vi "FPGA_Main.vi"() -> ()   [LabVIEW 2018]
uses:
  Data Def/FPGA_AI ADC IO.ctl
  Data Def/FPGA_AI ADC Loop Data.ctl
  Data Def/FPGA_AI ADC Loop State.ctl
  <vilib>/rvi/Emulation/niFpgaGetClockAttributes.vi
  <vilib>/rvi/Emulation/niFpgaSctlEmulationGetInTimedLoop.vi
  <vilib>/rvi/Emulation/niFpgaEmulationReportErrorSimple.vi
  <vilib>/rvi/Emulation/niFpgaCriticalErrorInLSC.vi
  SubVI/24AIO/AO/AO_FPGA.lvlib
panel:
  in  "AO_Data(U32)":u32
  out "C3 AI Data":i16[](array[numeric])
  out "C2 AI Data":i16[](array[numeric])
  out "C1 AI Data":i16[](array[numeric])
  out "C4 AI Data":i16[](array[numeric])
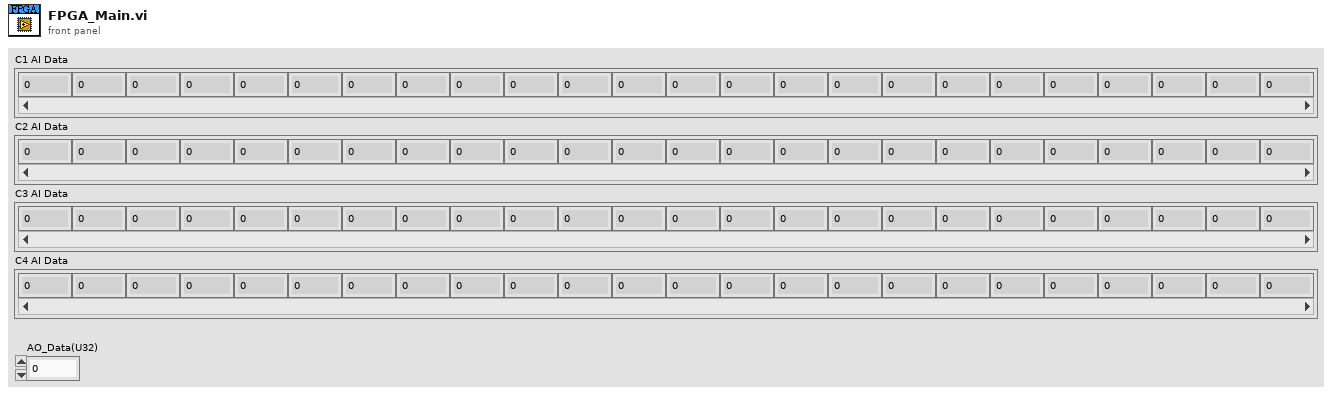
[diagram p1: front panel]
types:
  T1 = cluster{"CS":refnum<k21>, "CLK":refnum<k21>, "MOSI":refnum<k21>}
  T2 = typedef "FPGA_AI ADC IO.ctl" = cluster{"AI_A":cluster{"CONV":refnum<k21>, "RST":refnum<k21>, "SCK":refnum<k21>, "CS":refnum<k21>, "BUSY":refnum<k21>, "DOUT_A":refnum<k21>, "DOUT_B":refnum<k21>, "t_RST (ticks)":u32, "t_CONV (ticks)":u32, "t_BUSYMAX (ticks)":u32}, "AI_B":cluster{"CONV":refnum<k21>, "RST":refnum<k21>, "SCK":refnum<k21>, "CS":refnum<k21>, "BUSY":refnum<k21>, "DOUT_A":refnum<k21>, "DOUT_B":refnum<k21>, "t_RST (ticks)":u32, "t_CONV (ticks)":u32, "t_BUSYMAX (ticks)":u32}, "AI_C":cluster{"CONV":refnum<k21>, "RST":refnum<k21>, "SCK":refnum<k21>, "CS":refnum<k21>, "BUSY":refnum<k21>, "DOUT_A":refnum<k21>, "DOUT_B":refnum<k21>, "t_RST (ticks)":u32, "t_CONV (ticks)":u32, "t_BUSYMAX (ticks)":u32}}
  T3 = typedef "FPGA_AI ADC Loop Data.ctl" = cluster{"AI ADC Loop State":T4, "AI Data":i16[]}
  T4 = typedef "FPGA_AI ADC Loop State.ctl" = enum16{"Initialize", "Get Data"}
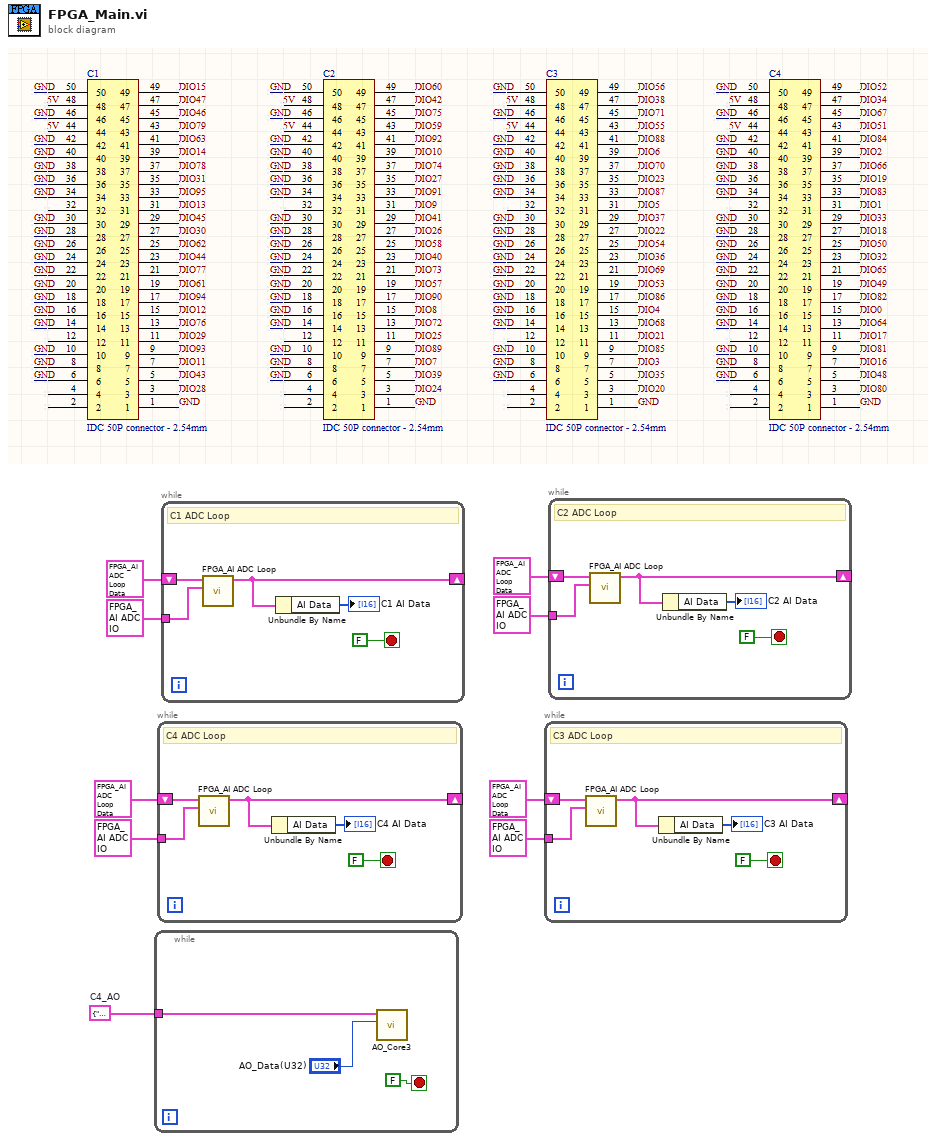
[diagram p0: block diagram]
diagram:
  w1 = T1 {"CS"="RMC/DIO67", "CLK"="RMC/DIO52", "MOSI"="RMC/DIO34"}  # C4_AO
  n1 = while {
    tunnel: w1 -> [w11]
    stop <- FALSE stop-if-true
    n2 = call "AO_Core3.vi"("data"="AO_Data(U32)", "Spi_A"=w11) -> ()  [unwired: 9 in, 1 out]
  }
  n3 = while {
    shift-right: [w17] -> _
    shift-left: T3 {"AI ADC Loop State"=enum."Initialize", "AI Data"=[0, 0, 0, 0, 0, 0, 0, 0, 0, 0, 0, 0, 0, 0, 0, 0, 0, 0, 0, 0, 0, 0, 0, 0]} ("AI ADC Loop Data") -> [w13]
    tunnel: T2 {"AI_A"={"CONV"="RMC/DIO0", "RST"="RMC/DIO64", "SCK"="RMC/DIO17", "CS"="RMC/DIO81", "BUSY"="RMC/DIO16", "DOUT_A"="RMC/DIO48", "DOUT_B"="RMC/DIO80", "t_RST (ticks)"=0, "t_CONV (ticks)"=0, "t_BUSYMAX (ticks)"=0}, "AI_B"={"CONV"="RMC/DIO33", "RST"="RMC/DIO18", "SCK"="RMC/DIO50", "CS"="RMC/DIO32", "BUSY"="RMC/DIO65", "DOUT_A"="RMC/DIO49", "DOUT_B"="RMC/DIO82", "t_RST (ticks)"=0, "t_CONV (ticks)"=0, "t_BUSYMAX (ticks)"=0}, "AI_C"={"CONV"="RMC/DIO51", "RST"="RMC/DIO84", "SCK"="RMC/DIO2", "CS"="RMC/DIO66", "BUSY"="RMC/DIO19", "DOUT_A"="RMC/DIO83", "DOUT_B"="RMC/DIO1", "t_RST (ticks)"=0, "t_CONV (ticks)"=0, "t_BUSYMAX (ticks)"=0}} ("AI ADC IO") -> [w14]
    stop <- FALSE stop-if-true
    # "C4 ADC Loop"
    n4 = call "FPGA_AI ADC Loop.vi"("AI ADC IO"=w14, "AI ADC Loop Data In"=w13) -> ("AI ADC Loop Data Out"=w17:T3)  [unwired: 9 in]
    n5 = Unbundle By Name(w17) -> ("AI Data"=→"C4 AI Data":i16[])
  }
  n6 = while {
    shift-right: [w22] -> _
    shift-left: T3 {"AI ADC Loop State"=enum."Initialize", "AI Data"=[0, 0, 0, 0, 0, 0, 0, 0, 0, 0, 0, 0, 0, 0, 0, 0, 0, 0, 0, 0, 0, 0, 0, 0]} ("AI ADC Loop Data") -> [w18]
    tunnel: T2 {"AI_A"={"CONV"="RMC/DIO12", "RST"="RMC/DIO76", "SCK"="RMC/DIO29", "CS"="RMC/DIO93", "BUSY"="RMC/DIO11", "DOUT_A"="RMC/DIO43", "DOUT_B"="RMC/DIO28", "t_RST (ticks)"=0, "t_CONV (ticks)"=0, "t_BUSYMAX (ticks)"=0}, "AI_B"={"CONV"="RMC/DIO45", "RST"="RMC/DIO30", "SCK"="RMC/DIO62", "CS"="RMC/DIO44", "BUSY"="RMC/DIO77", "DOUT_A"="RMC/DIO61", "DOUT_B"="RMC/DIO94", "t_RST (ticks)"=0, "t_CONV (ticks)"=0, "t_BUSYMAX (ticks)"=0}, "AI_C"={"CONV"="RMC/DIO79", "RST"="RMC/DIO63", "SCK"="RMC/DIO14", "CS"="RMC/DIO78", "BUSY"="RMC/DIO31", "DOUT_A"="RMC/DIO95", "DOUT_B"="RMC/DIO13", "t_RST (ticks)"=0, "t_CONV (ticks)"=0, "t_BUSYMAX (ticks)"=0}} ("AI ADC IO") -> [w19]
    stop <- FALSE stop-if-true
    # "C1 ADC Loop"
    n7 = call "FPGA_AI ADC Loop.vi"("AI ADC IO"=w19, "AI ADC Loop Data In"=w18) -> ("AI ADC Loop Data Out"=w22:T3)  [unwired: 9 in]
    n8 = Unbundle By Name(w22) -> ("AI Data"=→"C1 AI Data":i16[])
  }
  n9 = while {
    shift-right: [w27] -> _
    shift-left: T3 {"AI ADC Loop State"=enum."Initialize", "AI Data"=[0, 0, 0, 0, 0, 0, 0, 0, 0, 0, 0, 0, 0, 0, 0, 0, 0, 0, 0, 0, 0, 0, 0, 0]} ("AI ADC Loop Data") -> [w23]
    tunnel: T2 {"AI_A"={"CONV"="RMC/DIO4", "RST"="RMC/DIO68", "SCK"="RMC/DIO21", "CS"="RMC/DIO85", "BUSY"="RMC/DIO3", "DOUT_A"="RMC/DIO35", "DOUT_B"="RMC/DIO20", "t_RST (ticks)"=0, "t_CONV (ticks)"=0, "t_BUSYMAX (ticks)"=0}, "AI_B"={"CONV"="RMC/DIO37", "RST"="RMC/DIO22", "SCK"="RMC/DIO54", "CS"="RMC/DIO36", "BUSY"="RMC/DIO69", "DOUT_A"="RMC/DIO53", "DOUT_B"="RMC/DIO86", "t_RST (ticks)"=0, "t_CONV (ticks)"=0, "t_BUSYMAX (ticks)"=0}, "AI_C"={"CONV"="RMC/DIO55", "RST"="RMC/DIO88", "SCK"="RMC/DIO6", "CS"="RMC/DIO70", "BUSY"="RMC/DIO23", "DOUT_A"="RMC/DIO87", "DOUT_B"="RMC/DIO5", "t_RST (ticks)"=0, "t_CONV (ticks)"=0, "t_BUSYMAX (ticks)"=0}} ("AI ADC IO") -> [w24]
    stop <- FALSE stop-if-true
    # "C3 ADC Loop"
    n10 = call "FPGA_AI ADC Loop.vi"("AI ADC IO"=w24, "AI ADC Loop Data In"=w23) -> ("AI ADC Loop Data Out"=w27:T3)  [unwired: 9 in]
    n11 = Unbundle By Name(w27) -> ("AI Data"=→"C3 AI Data":i16[])
  }
  n12 = while {
    shift-right: [w32] -> _
    shift-left: T3 {"AI ADC Loop State"=enum."Initialize", "AI Data"=[0, 0, 0, 0, 0, 0, 0, 0, 0, 0, 0, 0, 0, 0, 0, 0, 0, 0, 0, 0, 0, 0, 0, 0]} ("AI ADC Loop Data") -> [w28]
    tunnel: T2 {"AI_A"={"CONV"="RMC/DIO8", "RST"="RMC/DIO72", "SCK"="RMC/DIO25", "CS"="RMC/DIO89", "BUSY"="RMC/DIO7", "DOUT_A"="RMC/DIO39", "DOUT_B"="RMC/DIO24", "t_RST (ticks)"=0, "t_CONV (ticks)"=0, "t_BUSYMAX (ticks)"=0}, "AI_B"={"CONV"="RMC/DIO41", "RST"="RMC/DIO26", "SCK"="RMC/DIO58", "CS"="RMC/DIO40", "BUSY"="RMC/DIO73", "DOUT_A"="RMC/DIO57", "DOUT_B"="RMC/DIO90", "t_RST (ticks)"=0, "t_CONV (ticks)"=0, "t_BUSYMAX (ticks)"=0}, "AI_C"={"CONV"="RMC/DIO59", "RST"="RMC/DIO92", "SCK"="RMC/DIO10", "CS"="RMC/DIO74", "BUSY"="RMC/DIO27", "DOUT_A"="RMC/DIO91", "DOUT_B"="RMC/DIO9", "t_RST (ticks)"=0, "t_CONV (ticks)"=0, "t_BUSYMAX (ticks)"=0}} ("AI ADC IO") -> [w29]
    stop <- FALSE stop-if-true
    # "C2 ADC Loop"
    n13 = call "FPGA_AI ADC Loop.vi"("AI ADC IO"=w29, "AI ADC Loop Data In"=w28) -> ("AI ADC Loop Data Out"=w32:T3)  [unwired: 9 in]
    n14 = Unbundle By Name(w32) -> ("AI Data"=→"C2 AI Data":i16[])
  }
